vi "PCSLauncher.contents.vi"   [LabVIEW 2014, in "PCSLauncher.lvlib"]
doc: "This class is forseen to control black boxes (motion).\n\nThis class is part of the PHELIX device layer."
uses:
  PCSLauncher.lvlib
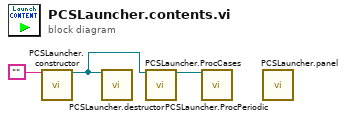
[diagram p0: block diagram]
diagram:
  n1 = call "PCSLauncher.constructor.vi"("name"="") -> ("i ref out"=w1:refnum<vi>)  [unwired: 16 in, 2 out]
  n2 = call "PCSLauncher.destructor.vi"("i ref in"=w1) -> ()  [unwired: 18 in, 1 out]
  n3 = call "PCSLauncher.ProcCases.vi"("i ref in"=w1) -> ("i ref out"=w2:refnum<vi>)  [unwired: 16 in, 2 out]
  n4 = call "PCSLauncher.ProcPeriodic.vi"("i ref in"=w2) -> ()  [unwired: 16 in, 3 out]
  n5 = call "PCSLauncher.panel.vi"() -> ()  [unwired: 19 in, 1 out]
